vi "Abort.vi"(8 "error in (no error)":errorcluster, 11 "AbortHandler in":refnum<class "SeqManager.lvclass">) -> (0 "error out":errorcluster, 3 "AbortHandler out":refnum<class "SeqManager.lvclass">)   [LabVIEW 2020, in "Volatus.lvlib" / "SeqManager.lvclass"]
uses:
  SeqManager.lvclass
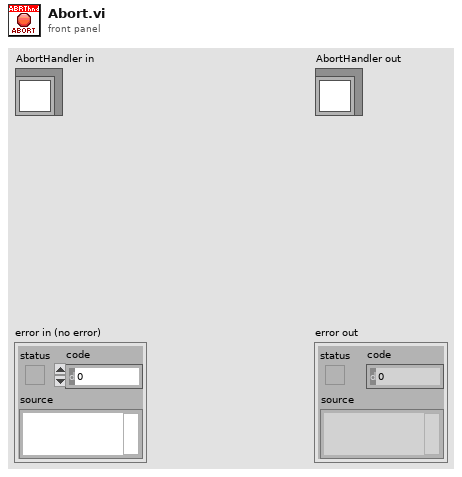
[diagram p1: front panel]
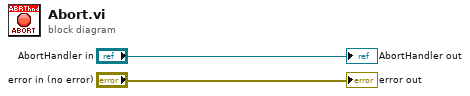
[diagram p0: block diagram]
diagram:
  "error out" <- "error in (no error)"
  "AbortHandler out" <- "AbortHandler in"
